vi "UTILITY Strip Increment Path.vi"(8 "Error In":errorcluster, 11 "file path in":path) -> (0 "Error Out":errorcluster, 3 "file path out":path)   [LabVIEW 2019]
uses:
  <vilib>/Utility/error.llb/whitespace.ctl
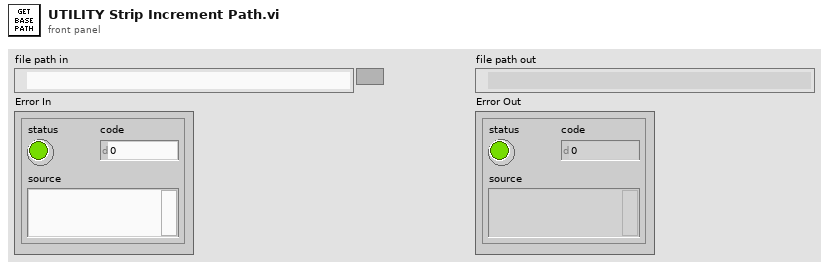
[diagram p1: front panel]
types:
  T1 = typedef "whitespace.ctl" = u16
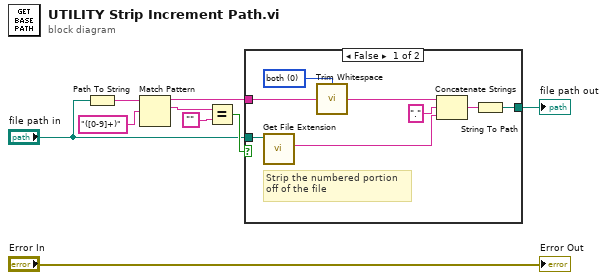
[diagram p0: block diagram]
diagram:
  n1 = Path To String(path="file path in") -> (string=w3:string)
  n2 = Match Pattern(string=w3, regular expression="([0-9]+)") -> (before substring=w5:string, match substring=w7:string)  [unwired: 1 in, 2 out]
  n3 = Equal?(x=w7, y="") -> (x = y?=w9:bool)
  n4 = case shown="False" w9 {
    tunnel: [w16 w18] -> w4
    tunnel: w5 -> [w15 _]
    tunnel: "file path in" -> [w14 w18]
    frame False {
      w17 = T1 0 items=["both", "start of string", "end of string"] ("location (both)")
      # "Strip the numbered portion\noff of the file"
      n5 = call <vilib>:"Get File Extension.vi"("file"=w14) -> ("lowercase file extension"=w11:string)  [unwired: 6 in, 4 out]
      n6 = call <vilib>:"Trim Whitespace.vi"("string"=w15, "location (both)"=w17) -> ("trimmed string"=w13:string)
      n7 = Concatenate Strings(w13, "." ("string"), w11) -> (w12:string)
      n8 = String To Path(string=w12) -> (path=w16:path)
    }
    frame True {
    }
  }
  "file path out" <- w4
  "Error Out" <- "Error In"
